vi "classes.vi"(0 "MoAgSy_Factory":refnum<class "MoAgSy_Factory.lvclass">, 1 "className":string, 5 "error in (no error)":errorcluster) -> (14 "MoAgSy_Factory dup":refnum<class "MoAgSy_Factory.lvclass">, 16 "Object":refnum<class>, 19 "error out":errorcluster)   [LabVIEW 2009, in "MoAgSy_Base.lvlib" / "MoAgSy_Factory.lvclass"]
doc: "This dynamaic dispatch VI contains constant objects of all classes that can be produced by HGF_Factory.\nClass has to be defined by name. \n\nOptionally, you can also specifiy a Class Path String instead, but you have to make sure that all dependencies are available.\n\nChild classes have to override it to define additional classes."
uses:
  MoAgSy_Factory.lvclass
  MoAgSy_Message/MoAgSy_Message.lvclass
  Visitors/MoAgSy_Visitor/MoAgSy_Visitor.lvclass
  Visitors/MoAgSy_Visitor_travel/MoAgSy_Visitor_travel.lvclass
  HGF_BaseClasses/HGF_Factory/HGF_Factory.lvclass
  MoAgSy_Engine/MoAgSy_Engine.lvclass
  MoAgSy_GPG/MoAgSy_GPG.lvclass
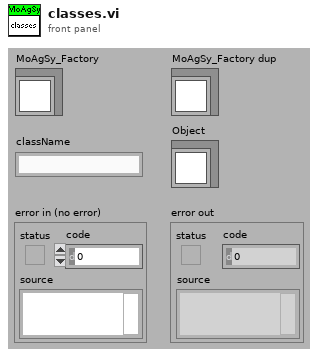
[diagram p1: front panel]
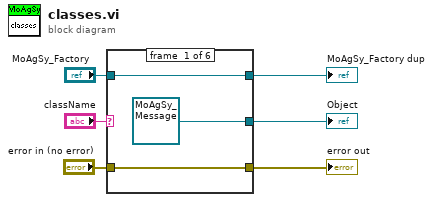
[diagram p0: block diagram]
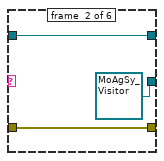
[diagram p2: hidden frame]
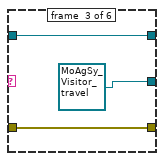
[diagram p3: hidden frame]
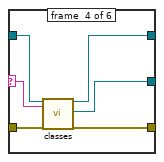
[diagram p4: hidden frame]
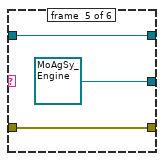
[diagram p5: hidden frame]
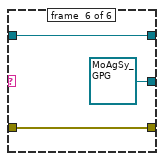
[diagram p6: hidden frame]
diagram:
  n1 = case shown="\"MoAgSy_Message\"" "className" {
    selector: "className" -> [_ _ _ w16 _ _]
    tunnel: "MoAgSy_Factory" -> [w9 w11 w14 w21 w23 w26]
    tunnel: "error in (no error)" -> [w8 w10 w13 w20 w22 w25]
    tunnel: [w9 w11 w14 w19 w23 w26] -> w4
    tunnel: [refnum<class "MoAgSy_Message.lvclass"> refnum ("MoAgSy.lvlib:MoAgSy_Message.lvclass") refnum<class "MoAgSy_Visitor.lvclass"> refnum ("MoAgSy.lvlib:MoAgSy_Visitor.lvclass") refnum<class "MoAgSy_Visitor_travel.lvclass"> refnum ("MoAgSy.lvlib:MoAgSy_Visitor_travel.lvclass") w18 refnum<class "MoAgSy_Engine.lvclass"> refnum ("MoAgSy.lvlib:MoAgSy_Engine.lvclass") refnum<class "MoAgSy_GPG.lvclass"> refnum ("MoAgSy.lvlib:MoAgSy_GPG.lvclass")] -> w3
    tunnel: [w8 w10 w13 w17 w22 w25] -> w2
    frame #0 {
    }
    frame #1 {
    }
    frame #2 {
    }
    frame #3 {
      n2 = call-parent "classes.vi"("HGF_Factory"=w21, "className"=w16, "error in (no error)"=w20) -> ("HGF_Factory dup"=w19:refnum<class "MoAgSy_Factory.lvclass">, "Object"=w18:refnum<class>, "error out"=w17:errorcluster)  [unwired: 14 out]
    }
    frame #4 {
    }
    frame #5 {
    }
  }
  "error out" <- w2
  "MoAgSy_Factory dup" <- w4
  "Object" <- w3
